vi "Get List of FPGAs From Monkey ID.vi"(8 "error in (no error)":errorcluster, 10 "Monkey ID":string, 11 "Tamer in":refnum<class "Tamer.lvclass">) -> (0 "error out":errorcluster, 1 "Monkey not found":bool, 2 "FPGA Names":string[](array[string]), 3 "Tamer out":refnum<class "Tamer.lvclass">)   [LabVIEW 2020, in "CIRCUS_uServices.lvlib" / "Tamer.lvlib" / "Tamer.lvclass"]
uses:
  Tamer.lvclass
  Tamer.lvclass/Tamer.ctl
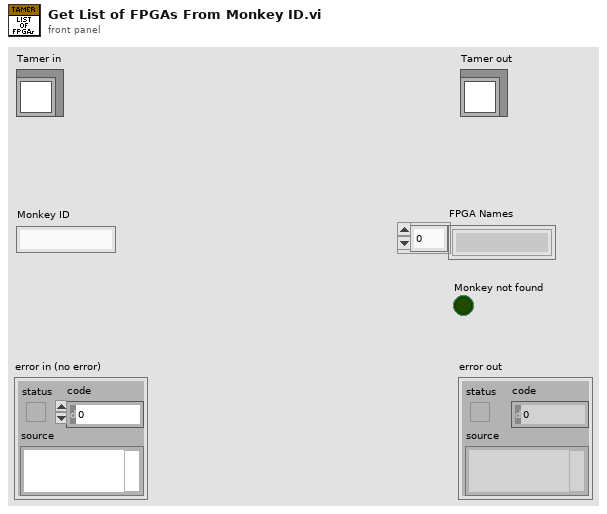
[diagram p1: front panel]
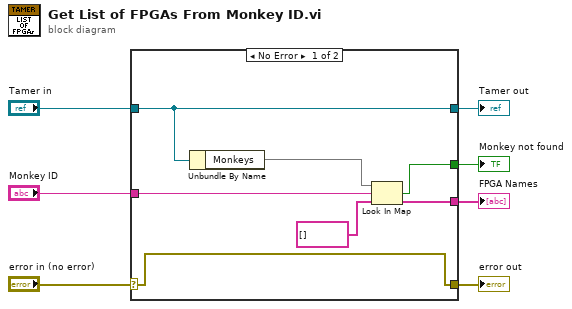
[diagram p0: block diagram]
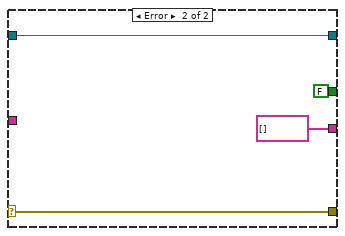
[diagram p2: hidden frame]
diagram:
  n1 = case shown="No Error" "error in (no error)" {
    selector: "error in (no error)" -> [w10 w18]
    tunnel: [w10 w18] -> w6
    tunnel: [w11 w17] -> w4
    tunnel: "Tamer in" -> [w11 w17]
    tunnel: "Monkey ID" -> [w13 _]
    tunnel: [w9 string[] [] ("Kasli Name")] -> w2
    tunnel: [w8 FALSE ("key not found?")] -> w1
    frame No Error {
      n2 = Unbundle By Name(w11) -> ("Monkeys"=w14:map{string, string[]})
      n3 = Look In Map(map=w14, key=w13, default value=string[] []) -> (key not found?=w8:bool, value=w9:string[])
    }
    frame Error {
    }
  }
  "error out" <- w6
  "Tamer out" <- w4
  "FPGA Names" <- w2
  "Monkey not found" <- w1
